vi "TagIDOutOfRangeError.vi"(8 "error in (no error)":errorcluster, 11 "Tag Family Size":i32) -> (0 "error out":errorcluster)   [LabVIEW 2020, in "feature_detection.lvlib"]
uses:
  feature_detection.lvlib
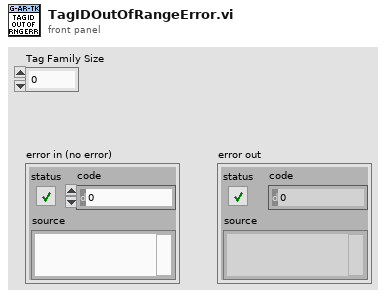
[diagram p1: front panel]
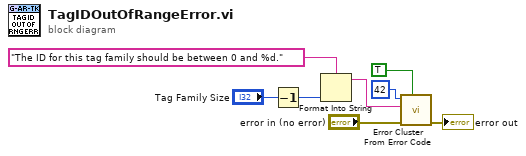
[diagram p0: block diagram]
diagram:
  n1 = Decrement(x="Tag Family Size") -> (x-1=w1:i32)
  n2 = Format Into String(format string="The ID for this tag family should be between 0 and %d.", w1) -> (resulting string=w4:string)  [unwired: 2 in, 1 out]
  n3 = call <vilib>:"Error Cluster From Error Code.vi"("show call chain? (False)"=TRUE, "error in (no error)"="error in (no error)", "error message (\"\")"=w4, "error code (0)"=42) -> ("error out"=→"error out":errorcluster)  [unwired: 5 in]
